vi "IsIOAlias.vi"(8 "error in (no error)":errorcluster, 11 "project var in":refnum<vi>) -> (0 "error out":errorcluster, 2 "is io var?":bool, 3 "project var out":refnum<vi>)   [LabVIEW 2020]
uses:
  <vilib>/variable/NI_Variable.lvlib
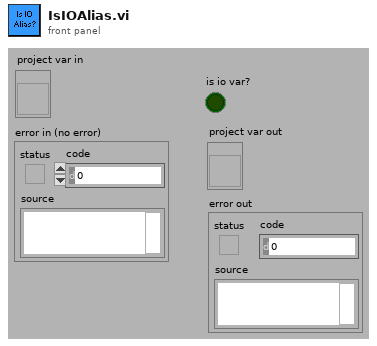
[diagram p1: front panel]
types:
  T1 = enum16{"Single-Process", "Network-Published", "Time-Triggered", "Industrial"}
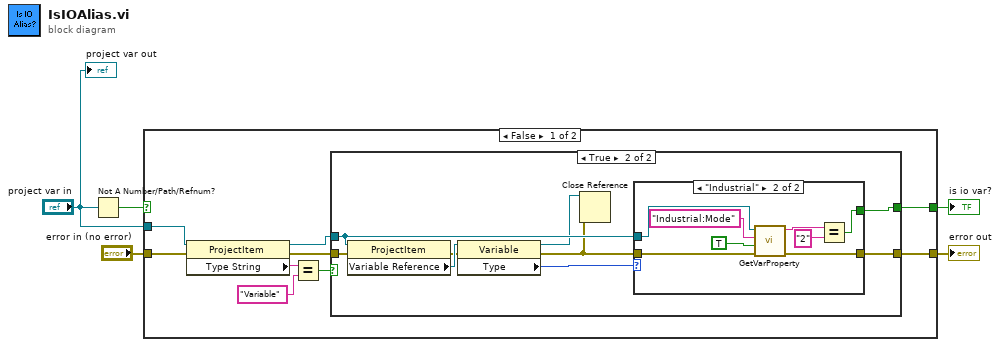
[diagram p0: block diagram]
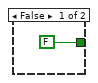
[diagram p2: hidden frame]
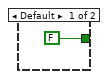
[diagram p3: hidden frame]
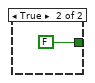
[diagram p4: hidden frame]
diagram:
  n1 = Not A Number/Path/Refnum?(number/path/refnum="project var in") -> (NaN/Path/Refnum?=w4:bool)
  n2 = case shown="False" w4 {
    tunnel: [w14 FALSE] -> w5
    tunnel: "project var in" -> [w13 _]
    tunnel: [w7 _] -> w2
    tunnel: "error in (no error)" -> [w6 _]
    frame False {
      n3 = property class="ProjectItem"(reference=w13, error in=w6) -> (reference out=w12:refnum<vi>, error out=w8:errorcluster, "Type String"=w11:string)
      n4 = Equal?(x=w11, y="Variable") -> (x = y?=w9:bool)
      n5 = case shown="True" w9 {
        tunnel: [FALSE w23] -> w14
        tunnel: w12 -> [_ w18]
        tunnel: w8 -> [_ w20]
        tunnel: [_ w19] -> w7
        frame False {
        }
        frame True {
          n6 = property class="ProjectItem"(reference=w18, error in=w20) -> (error out=w21:errorcluster, "Variable Reference"=w22:refnum<vi>)  [unwired: 1 out]
          n7 = property class="Variable"(reference=w22, error in=w21) -> (reference out=w17:refnum<vi>, error out=w16:errorcluster, "Type"=w24:T1)
          n8 = Close Reference(reference=w17, error in (no error)=w16) -> ()  [unwired: 1 out]
          n9 = case shown="\"Industrial\"" w24 {
            tunnel: [FALSE w33] -> w23
            tunnel: w18 -> [_ w31]
            tunnel: w16 -> [_ w29]
            tunnel: [_ w26] -> w19
            frame Default {
            }
            frame "Industrial" {
              n10 = call <vilib>:"GetVarProperty.vi"("error in (no error)"=w29, "use namespace bag?"=TRUE, "property name in"="Industrial:Mode", "project var in"=w31) -> ("error out"=w26:errorcluster, "property value out"=w27:string)  [unwired: 6 out]
              n11 = Equal?(x=w27, y="2") -> (x = y?=w33:bool)
            }
          }
        }
      }
    }
    frame True {
    }
  }
  "is io var?" <- w5
  "error out" <- w2
  "project var out" <- "project var in"
